vi "PCO_Config.vi"(5 "ExposureTimeBase":u16(ring)=2 items=["nanoseconds", "microseconds", "milliseconds"], 7 "Exposure":u32=10, 8 "ErrorIn":errorcluster, 11 "ph":u64) -> (0 "error out":errorcluster, 3 "hout":u64)   [LabVIEW 2011]
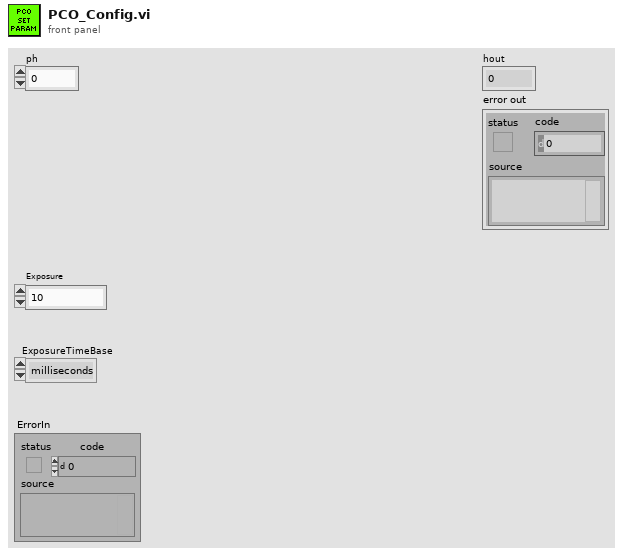
[diagram p1: front panel]
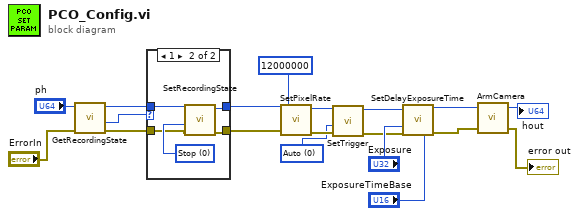
[diagram p0: block diagram]
diagram:
  w13 = u16 0 items=["Auto", "Software", "External sequence start ", "External exposure control"] ("TriggerMode")
  n1 = call <userlib>:"GetRecordingState.vi"("ErrorIn"="ErrorIn", "ph"="ph") -> ("ErrorOut"=w12:errorcluster, "RecordingState"=w10:u16, "hout"=w11:u64)  [unwired: 2 in, 1 out]
  n2 = case shown="1" w10 {
    tunnel: w11 -> [w21 w25]
    tunnel: w12 -> [w20 w24]
    tunnel: [w21 w23] -> w8
    tunnel: [w20 w22] -> w7
    frame 0, Default {
    }
    frame 1 {
      w26 = u16 0 items=["Stop", "Run"] ("RecordingState")
      n3 = call <userlib>:"SetRecordingState.vi"("ErrorIn"=w24, "RecordingState"=w26, "ph"=w25) -> ("ErrorOut"=w22:errorcluster, "hout"=w23:u64)  [unwired: 2 in, 1 out]
    }
  }
  n4 = call <userlib>:"SetPixelRate.vi"("error in (no error)"=w7, "PixelRate"=u32 12000000, "ph"=w8) -> ("error out"=w19:errorcluster, "hout"=w18:u64)  [unwired: 2 in, 1 out]
  n5 = call <userlib>:"SetTrigger.vi"("error in (no error)"=w19, "TriggerMode"=w13, "ph"=w18) -> ("error out"=w15:errorcluster, "hout"=w14:u64)  [unwired: 2 in, 1 out]
  n6 = call <userlib>:"SetDelayExposureTime.vi"("ph"=w14, "Exposure"="Exposure", "error in (no error)"=w15, "ExposureTimeBase"="ExposureTimeBase") -> ("hout"=w5:u64, "error out"=w4:errorcluster)  [unwired: 9 in, 1 out]
  n7 = call <userlib>:"ArmCamera.vi"("error in (no error)"=w4, "ph"=w5) -> ("error out"=→"error out":errorcluster, "hout"=→"hout":u64)  [unwired: 1 in, 1 out]
